vi "HAPS_main_Phase_Cali_Preamp.vi"() -> ()   [LabVIEW 2023, in "HAPS.lvlib"]
uses:
  HAPS.lvlib
  MCU_Function.ctl
  set_ele.ctl
  HAPS_SerialPort.ctl
  HAPS_MCU_ELE_Func.ctl
panel:
  in  "FileNote":string
  out "Array 2":dbl[](array[numeric])
  out "Array":i32[](array[numeric])
  out "ele_gain":i32
  out "comn_gain":i32
  out "Duration":dbl
  in  "Init?":bool
  out "In-Phase : Phase(degree)":dbl[](graph)
  out "In-Phase : Gain(dB)":dbl[](graph)
  out "channel":i32
  out "chain_id":i32
  out "group":i32
  out "array_id":i32
  in  "Phase diff. Criteria":dbl format="%#_13g"
  in  "Tx/Rx":enum16{"Rx", "Tx"}(ring)=enum."Tx"
  in  "array_id (MCU index)":i32
  in  "MCU_UART_addr":refnum<visa-resource-name>="COM1"
  in  "Max Steps":i32=10
  in  "Target(degree)":dbl format="%#_13g"
  in  "SweepPoints":i32=11
  in  "sParameter":i32=21
  in  "Stop_Freq(GHz)":dbl=39.5
  in  "Start_Freq(GHz)":dbl=38.5
  in  "VISA resource name":refnum<visa-resource-name>="TCPIP0::192.168.119.45::inst0::INSTR"
  in  "HAPS_Equipment":enum16{"Keysight", "R&S"}(ring)=enum."R&S"
  # "TCPIP0::169.254.52.242::hislip0::INSTR"
  # "TCPIP0::192.168.119.45::inst0::INSTR"
  # "HAPS_24x24_Phase_Calibration_Preamp"
  # "VNA"
  # "TCPIP0::192.168.1.31::hislip0::INSTR"
  # "Test Status"
  # "DUT"
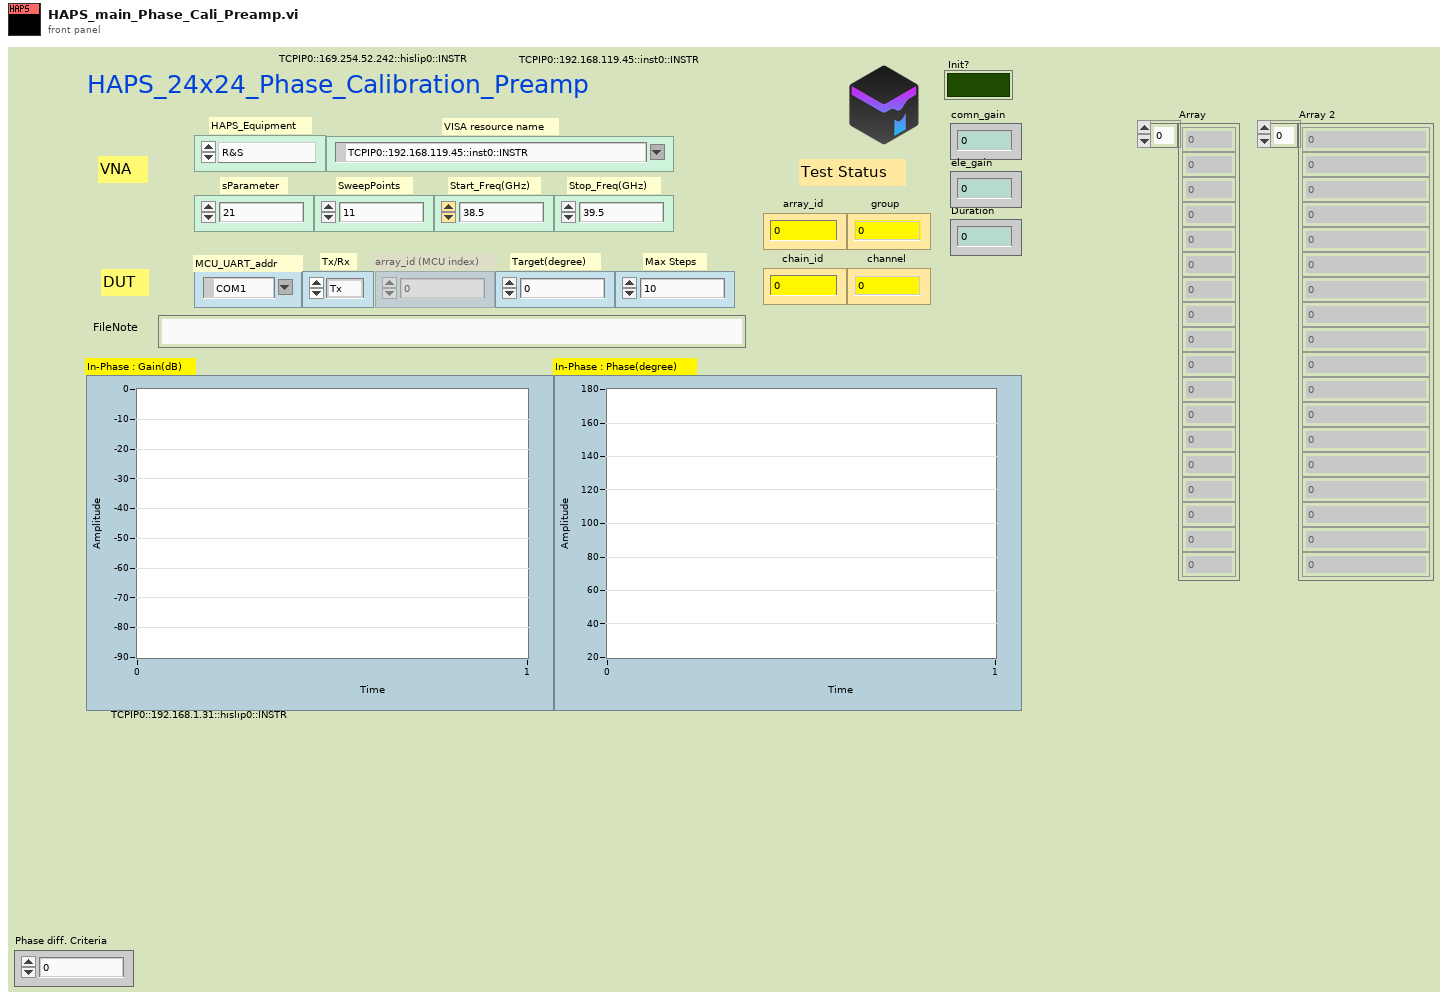
[diagram p1: front panel]
types:
  T1 = typedef "HAPS.lvlib/HAPS_SerialPort.ctl" = enum16{"Init", "Close", "CMD", "Flush"}
  T2 = typedef "HAPS.lvlib/HAPS_MCU_ELE_Func.ctl" = enum16{"array_init", "set_com_gain", "set_ch_gain_phase", "set_pd_range", "get_preamp_temp", "get_bfic_temp", "get_tx_pd", "ch_on", "ch_on_2", "ch_ctrl_all", "array_ctrl_src"}
  T3 = typedef "HAPS.lvlib/set_ele.ctl" = cluster{"ch":i32, "chain_id":i32, "group":i32, "array_id":i32, "ele_phase":i32, "ele_gain":i32, "com_gain":i32, "pd_range":i32}
  T4 = typedef "HAPS.lvlib/MCU_Function.ctl" = cluster{"Tx/Rx":enum16{"Rx", "Tx"}, "Enable?":enum16{"OFF", "On"}, "Source":enum16{"MCU", "ACU"}}
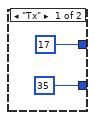
[diagram p2: hidden frame]
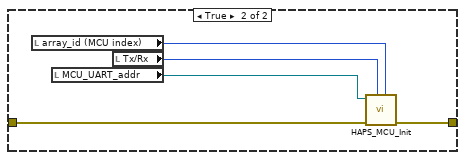
[diagram p3: hidden frame]
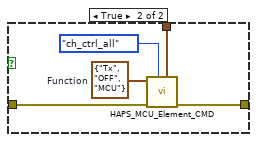
[diagram p6: hidden frame]
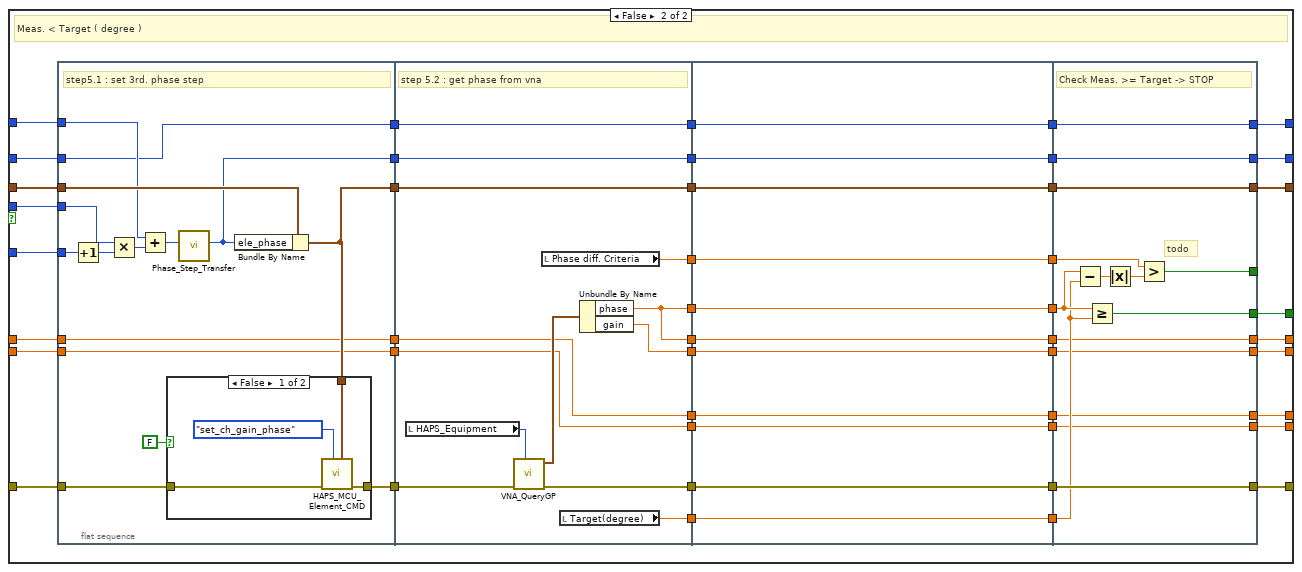
[diagram p11: hidden frame]
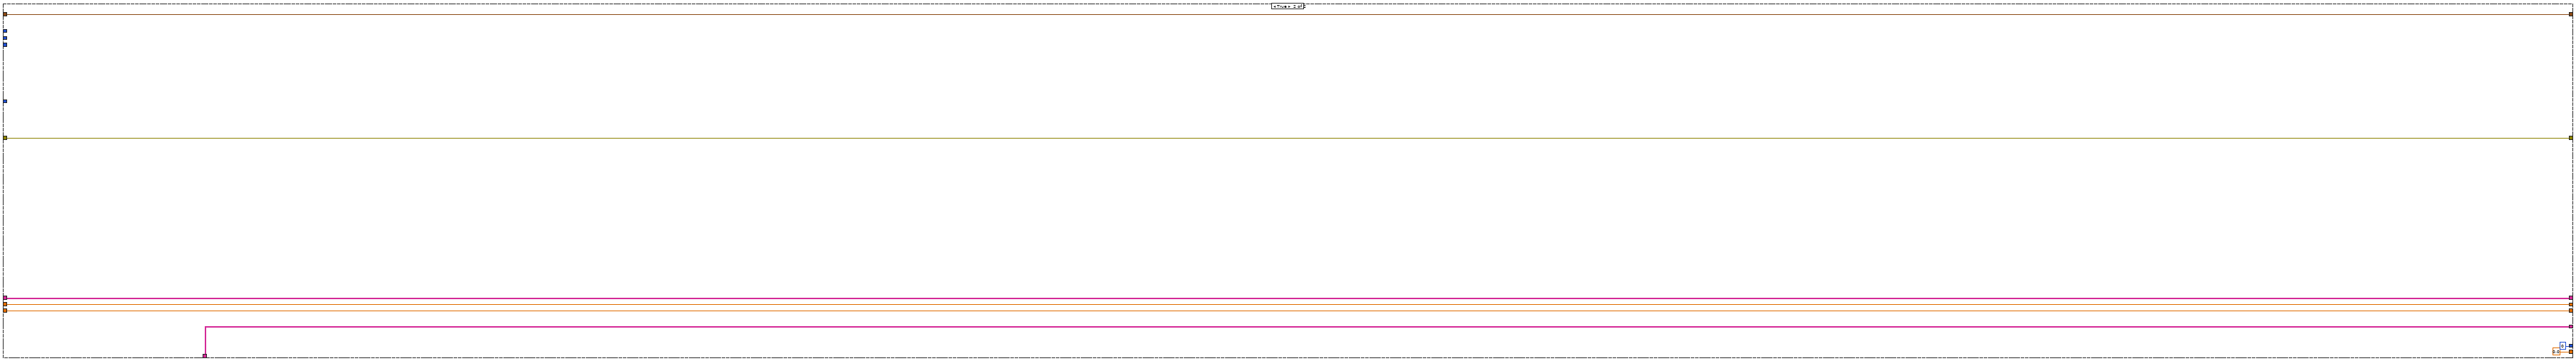
[diagram p13: hidden frame]
diagram:
  n1 = flat-sequence {
    tunnel: [w23] -> w16
    tunnel: [w30] -> w15
    tunnel: [errorcluster {"status"=FALSE, "code"=0, "source"=""} ("error in")] -> w13
    tunnel: ["sParameter"] -> w11
    tunnel: ["VISA resource name"] -> w10
    tunnel: ["Start_Freq(GHz)"] -> w9
    tunnel: ["Stop_Freq(GHz)"] -> w8
    tunnel: ["SweepPoints"] -> w7
    tunnel: ["HAPS_Equipment"] -> w6
    tunnel: [w20] -> w4
    tunnel: w16 -> [w47]
    tunnel: w15 -> [_]
    tunnel: [w47] -> w14
    tunnel: w13 -> [w46]
    tunnel: [w38] -> w12
    tunnel: w11 -> [w45]
    tunnel: w10 -> [w44]
    tunnel: w9 -> [w43]
    tunnel: w8 -> [w42]
    tunnel: w7 -> [w41]
    tunnel: w6 -> [w37]
    tunnel: [w35] -> w5
    tunnel: w4 -> [w35]
    tunnel: w14 -> [w67]
    tunnel: w12 -> [w68]
    tunnel: w5 -> [w64]
    tunnel: [w64] -> w3
    tunnel: [w63] -> w2
    tunnel: [w61] -> w1
    tunnel: [w631] -> _
    tunnel: w3 -> [w631]
    tunnel: w2 -> [w633]
    tunnel: w1 -> [w623]
    frame #0 {
      w21 = dbl[] []
      w23 = T3 {"ch"=0, "chain_id"=0, "group"=0, "array_id"=0, "ele_phase"=0, "ele_gain"=0, "com_gain"=0, "pd_range"=0}  # set_ele
      w30 = T4 {"Tx/Rx"=enum."Tx", "Enable?"=enum."OFF", "Source"=enum."MCU"}  # Function
      # "Init"
      n2 = case shown="\"Rx\"" "Tx/Rx" {
        tunnel: [17 ("comn_ele_gain") 17 ("comn_ele_gain")] -> w18
        tunnel: [35 ("comn_ele_gain") 22 ("comn_ele_gain")] -> w17
        frame "Tx" {
        }
        frame "Rx" {
        }
      }
      "comn_gain" <- w18
      "ele_gain" <- w17
      n3 = Get Date/Time In Seconds() -> (seconds since 1Jan1904=w20:timestamp)
      "In-Phase : Gain(dB)" <- w21
      "In-Phase : Phase(degree)" <- w21
    }
    frame #1 {
      # "settting before Calibration"
      n4 = call "VNA_init.vi"("Stop_Freq(GHz)"=w42, "HAPS_MCU_CMD"=w37, "Start_Freq(GHz)"=w43, "sParameter"=w45, "error in"=w46, "SweepPoints"=w41, "Mark no."=1, "VISA resource name"=w44) -> ("error out"=w39:errorcluster)  [unwired: 3 in]
      n5 = case shown="False" "Init?" {
        tunnel: w39 -> [w54 w59]
        tunnel: [w50 w58] -> w38
        frame False {
          n6 = local read "MCU_UART_addr"() -> (w52:refnum<visa-resource-name>)
          n7 = call "HAPS_MCU_SerialPort.vi"("HAPS_SerialPort_Func"=HAPS_SerialPort."Init", "error in"=w54, "VISA resource name"=w52) -> ("error out"=w51:errorcluster)  [unwired: 6 in, 2 out]
          n8 = call "HAPS_MCU_SerialPort.vi"("Command"="log_en 0", "HAPS_SerialPort_Func"=enum16{"Init", "Close", "CMD"}."CMD" ("HAPS_SerialPort"), "error in"=w51) -> ("error out"=w50:errorcluster)  [unwired: 6 in, 2 out]
        }
        frame True {
          n9 = local read "array_id (MCU index)"() -> (w56:i32)
          n10 = local read "MCU_UART_addr"() -> (w57:refnum<visa-resource-name>)
          n11 = local read "Tx/Rx"() -> (w55:enum16{"Rx", "Tx"})
          n12 = call "HAPS_MCU_Init.vi"("array_id"=w56, "Tx/Rx"=w55, "error in"=w59, "VISA resource name"=w57) -> ("error out"=w58:errorcluster)  [unwired: 7 in]
        }
      }
    }
    frame #2 {
      w60 = i32[][] [[2, 0, 0, 8, 8, 10, 11, 9, 9, 1, 1, 3], [3, 1, 1, 9, 9, 11, 13, 15, 15, 7, 7, 5], [5, 7, 7, 15, 15, 13, 14, 14, 6, 6, 4, 12]]  # Preamp_ch
      # "Calibration"
      n13 = for {
        N: 3 -> [_]
        shift-right: [w79] -> _
        shift-left: w67 -> [w75]
        shift-right: [w78] -> w63
        shift-left: string[][] [] -> [w73]
        shift-right: [w77] -> _
        shift-left: w68 -> [w76]
        shift-right: [w71] -> w61
        shift-left: string[][] [] -> [w72]
        tunnel: w60 -> [w70] mode=indexing
        i -> [w74]
        w69 = dbl[] []
        # "group ( 0~2 )"
        n14 = for {
          N: 12 -> [_]
          shift-right: [w95] -> w79
          shift-left: w75 -> [w91]
          shift-right: [w94] -> w78
          shift-left: w73 -> [w88]
          shift-right: [w93] -> w77
          shift-left: w76 -> [w92]
          tunnel: w74 -> [w90]
          shift-right: [w83] -> _
          shift-left: w69 -> [_]
          shift-right: [w83] -> _
          shift-left: w69 -> [_]
          shift-right: [w86] -> w71
          shift-left: w72 -> [w87]
          tunnel: w70 -> [w85] mode=indexing
          i -> [w89]
          w83 = dbl[] []
          w84 = dbl[] []
          # "Chain_id ( 0~11 )"
          n15 = for {
            N: 16 -> [_]
            shift-right: [w119] -> w95
            shift-left: w91 -> [w107]
            shift-right: [w117] -> w94
            shift-left: w88 -> [w118]
            shift-right: [w109] -> w93
            shift-left: w92 -> [w108]
            tunnel: w90 -> [w101]
            tunnel: w89 -> [w100]
            shift-right: [w114] -> _
            shift-left: w84 -> [w116]
            shift-right: [w113] -> _
            shift-left: w84 -> [w115]
            shift-right: [w111] -> w86
            shift-left: w87 -> [w112]
            tunnel: w85 -> [w106]
            tunnel: [w98] -> w82 mode=indexing
            tunnel: [w97] -> w81 mode=indexing
            i -> [w110]
            # "Channel ( 0~15 )"
            n16 = Equal?(x=2, y=w101) -> (x = y?=w105:bool)
            n17 = Equal?(x=11, y=w100) -> (x = y?=w104:bool)
            n18 = And(x=w105, y=w104) -> (x .and. y?=w99:bool)
            n19 = case shown="False" w99 {
              tunnel: [w120 w615] -> w119
              tunnel: w118 -> [w152 w617]
              tunnel: [w151 w617] -> w117
              tunnel: w116 -> [w150 w618]
              tunnel: w115 -> [w149 w619]
              tunnel: [w148 w618] -> w114
              tunnel: [w147 w619] -> w113
              tunnel: w112 -> [w146 w620]
              tunnel: [w145 w620] -> w111
              tunnel: w101 -> [w128 _]
              tunnel: w100 -> [w127 _]
              tunnel: w110 -> [w142 _]
              tunnel: [w140 w616] -> w109
              tunnel: w108 -> [w136 w616]
              tunnel: w107 -> [w134 w615]
              tunnel: w106 -> [w129 _]
              tunnel: [w122 0 ("Esitmation_Step")] -> w98
              tunnel: [w121 0.0 ("phase")] -> w97
              frame False {
                n20 = local read "array_id (MCU index)"() -> (w132:i32)
                n21 = Bundle By Name(cluster=w134, "array_id"=w132, "group"=3, "chain_id"=0, "ch"=w129) -> (w133:T3)
                n22 = call "HAPS_MCU_Element_CMD.vi"("set_ele"=w133, "HAPS_MCU_ELE_Func."=HAPS_MCU_ELE_Func."ch_on", "error in"=w136) -> ("error out"=w135:errorcluster)  [unwired: 7 in, 1 out]
                n23 = Bundle By Name(cluster=w134, "array_id"=w132, "group"=w128, "chain_id"=w127, "ch"=w142) -> (w141:T3)
                n24 = call "HAPS_MCU_Element_CMD.vi"("set_ele"=w141, "HAPS_MCU_ELE_Func."=HAPS_MCU_ELE_Func."ch_on", "error in"=w135) -> ("error out"=w143:errorcluster)  [unwired: 7 in, 1 out]
                n25 = flat-sequence {
                  tunnel: w141 -> [w229]
                  tunnel: w143 -> [w230]
                  tunnel: [w231] -> w207
                  tunnel: [w227] -> w206
                  tunnel: w142 -> [w226]
                  tunnel: [w225] -> w205
                  tunnel: w152 -> [w225]
                  tunnel: w128 -> [w223]
                  tunnel: w127 -> [w222]
                  tunnel: [w221] -> w204
                  tunnel: w150 -> [w221]
                  tunnel: [w220] -> w203
                  tunnel: w149 -> [w220]
                  tunnel: w146 -> [w219]
                  tunnel: [w219] -> w202
                  tunnel: w207 -> [w248]
                  tunnel: [w249] -> w201
                  tunnel: [w240] -> w200
                  tunnel: [w247] -> w199
                  tunnel: w206 -> [w247]
                  tunnel: [w244] -> w198
                  tunnel: w205 -> [w244]
                  tunnel: [w243] -> w197
                  tunnel: w204 -> [w243]
                  tunnel: [w242] -> w196
                  tunnel: w203 -> [w242]
                  tunnel: w202 -> [w241]
                  tunnel: [w241] -> w195
                  tunnel: [w240] -> w122
                  tunnel: [w239] -> w121
                  tunnel: w201 -> [w254]
                  tunnel: [w255] -> w194
                  tunnel: w200 -> [w260]
                  tunnel: [w260] -> w193
                  tunnel: w199 -> [w253]
                  tunnel: [w253] -> w192
                  tunnel: w198 -> [w259]
                  tunnel: [w259] -> w191
                  tunnel: w197 -> [w258]
                  tunnel: [w258] -> w190
                  tunnel: w196 -> [w257]
                  tunnel: [w257] -> w189
                  tunnel: w195 -> [w256]
                  tunnel: [w256] -> w188
                  tunnel: w194 -> [w275]
                  tunnel: w193 -> [w272]
                  tunnel: w192 -> [w274]
                  tunnel: [w276] -> w187
                  tunnel: [w273] -> w186
                  tunnel: [w272] -> w185
                  tunnel: [w271] -> w184
                  tunnel: w191 -> [w271]
                  tunnel: w190 -> [w270]
                  tunnel: w189 -> [w269]
                  tunnel: [w270] -> w183
                  tunnel: [w269] -> w182
                  tunnel: w188 -> [w268]
                  tunnel: [w268] -> w181
                  tunnel: w187 -> [w297]
                  tunnel: w186 -> [w290]
                  tunnel: [w298] -> w180
                  tunnel: [w292] -> w179
                  tunnel: [w291] -> w178
                  tunnel: [w290] -> w177
                  tunnel: [w289] -> w176
                  tunnel: w185 -> [w289]
                  tunnel: [w287] -> w175
                  tunnel: w184 -> [w287]
                  tunnel: [w286] -> w174
                  tunnel: w183 -> [w286]
                  tunnel: [w285] -> w173
                  tunnel: w182 -> [w285]
                  tunnel: w181 -> [w284]
                  tunnel: [w284] -> w172
                  tunnel: [w283] -> w126
                  tunnel: [w282] -> w124
                  tunnel: w180 -> [w302]
                  tunnel: [w303] -> w171
                  tunnel: w179 -> [w311]
                  tunnel: [w311] -> w170
                  tunnel: w178 -> [w310]
                  tunnel: [w310] -> w169
                  tunnel: w177 -> [w309]
                  tunnel: [w309] -> w168
                  tunnel: w176 -> [w308]
                  tunnel: [w308] -> w167
                  tunnel: w175 -> [w307]
                  tunnel: [w307] -> w166
                  tunnel: w174 -> [w306]
                  tunnel: [w306] -> w165
                  tunnel: w173 -> [w305]
                  tunnel: [w305] -> w164
                  tunnel: w172 -> [w304]
                  tunnel: [w304] -> w163
                  tunnel: w126 -> [w300]
                  tunnel: [w300] -> w125
                  tunnel: w124 -> [w299]
                  tunnel: [w299] -> w123
                  tunnel: w171 -> [w331]
                  tunnel: w170 -> [w332]
                  tunnel: w169 -> [w333]
                  tunnel: w168 -> [w334]
                  tunnel: w167 -> [w319]
                  tunnel: [w330] -> w162
                  tunnel: [w329] -> w161
                  tunnel: [w328] -> w160
                  tunnel: [w327] -> w159
                  tunnel: [w326] -> w158
                  tunnel: [w325] -> w157
                  tunnel: w166 -> [w325]
                  tunnel: [w324] -> w156
                  tunnel: w165 -> [w323]
                  tunnel: w164 -> [w322]
                  tunnel: [w323] -> w155
                  tunnel: [w322] -> w154
                  tunnel: w163 -> [w321]
                  tunnel: [w320] -> w153
                  tunnel: w125 -> [w318]
                  tunnel: w123 -> [w317]
                  tunnel: [w612] -> w120
                  tunnel: w162 -> [w612]
                  tunnel: w161 -> [w611]
                  tunnel: w160 -> [w583]
                  tunnel: w159 -> [w584]
                  tunnel: w158 -> [w606]
                  tunnel: w157 -> [w590]
                  tunnel: [w592] -> w151
                  tunnel: [w591] -> w139
                  tunnel: w156 -> [w591]
                  tunnel: w155 -> [w587]
                  tunnel: w154 -> [w586]
                  tunnel: [w589] -> w148
                  tunnel: [w588] -> w147
                  tunnel: w153 -> [w582]
                  tunnel: [w582] -> w145
                  frame #0 {
                    w232 = 0  # pd_range
                    w233 = 0  # Init_Phase_Step
                    # "step 1. : First get phase step \"0\" for element BFIC"
                    n26 = local read "array_id (MCU index)"() -> (w224:i32)
                    "array_id" <- w224
                    n27 = local read "ele_gain"() -> (w216:i32)
                    n28 = local read "comn_gain"() -> (w217:i32)
                    n29 = Bundle By Name(cluster=w229, "array_id"=w224, "group"=w223, "chain_id"=w222, "ch"=w226, "com_gain"=w217, "ele_gain"=w216, "ele_phase"=w233, "pd_range"=w232) -> (w227:T3)
                    n30 = case shown="False" FALSE {
                      tunnel: [w237 w238] -> w231
                      tunnel: w230 -> [w236 w238]
                      tunnel: HAPS_MCU_ELE_Func."set_ch_gain_phase" ("HAPS_MCU_ELE_Func.") -> [w235 _]
                      tunnel: w227 -> [w234 _]
                      frame False {
                        n31 = call "HAPS_MCU_Element_CMD.vi"("set_ele"=w234, "HAPS_MCU_ELE_Func."=w235, "error in"=w236) -> ("error out"=w237:errorcluster)  [unwired: 7 in, 1 out]
                      }
                      frame True {
                      }
                    }
                    "group" <- w223
                    "chain_id" <- w222
                    "channel" <- w226
                  }
                  frame #1 {
                    # "todo:gain"
                    # "step 2. : get first pahse data from vna"
                    n32 = local read "HAPS_Equipment"() -> (w245:enum16{"Keysight", "R&S"})
                    n33 = call "VNA_QueryGP.vi"("HAPS_Equipment"=w245, "error in"=w248) -> ("error out"=w249:errorcluster, "queryMarker"=w250:cluster{"gain":dbl, "phase":dbl})  [unwired: 8 in]
                    n34 = Unbundle By Name(w247) -> ("ele_phase"=w246:i32)
                    n35 = local read "Target(degree)"() -> (w251:dbl)
                    n36 = Unbundle By Name(w250) -> ("phase"=w239:dbl)  [unwired: 1 out]
                    n37 = call "Estimation_Steps.vi"("Target(degree)"=w251, "Source_Phase_Step"=w246, "Input_Phase(degree)"=w239) -> ("Esitmation_Step"=w240:i32)  [unwired: 7 in, 1 out]
                  }
                  frame #2 {
                    n38 = case shown="False" FALSE {
                      tunnel: [w261 w266] -> w255
                      tunnel: w254 -> [w261 w265]
                      tunnel: w253 -> [_ w263]
                      frame False {
                      }
                      frame True {
                        w262 = T4 {"Tx/Rx"=enum."Tx", "Enable?"=enum."OFF", "Source"=enum."MCU"}  # Function
                        n39 = call "HAPS_MCU_Element_CMD.vi"("set_ele"=w263, "HAPS_MCU_ELE_Func."=HAPS_MCU_ELE_Func."ch_ctrl_all", "error in"=w265, "Function"=w262) -> ("error out"=w266:errorcluster)  [unwired: 6 in, 1 out]
                      }
                    }
                  }
                  frame #3 {
                    # "source.\nphase step"
                    # "step 3.  set estimation phase step in second time"
                    n40 = Bundle By Name(cluster=w274, "ele_phase"=w272) -> (w273:T3)
                    n41 = case shown="False" FALSE {
                      tunnel: [w280 w281] -> w276
                      tunnel: w275 -> [w279 w281]
                      tunnel: w273 -> [w278 _]
                      frame False {
                        n42 = call "HAPS_MCU_Element_CMD.vi"("set_ele"=w278, "HAPS_MCU_ELE_Func."=HAPS_MCU_ELE_Func."set_ch_gain_phase", "error in"=w279) -> ("error out"=w280:errorcluster)  [unwired: 7 in, 1 out]
                      }
                      frame True {
                      }
                    }
                  }
                  frame #4 {
                    # "todo:gain"
                    # "step 4. : get second time pahse from vna"
                    n43 = local read "HAPS_Equipment"() -> (w288:enum16{"Keysight", "R&S"})
                    n44 = call "VNA_QueryGP.vi"("HAPS_Equipment"=w288, "error in"=w297) -> ("error out"=w298:errorcluster, "queryMarker"=w293:cluster{"gain":dbl, "phase":dbl})  [unwired: 8 in]
                    n45 = Unbundle By Name(w293) -> ("phase"=w283:dbl, "gain"=w282:dbl)
                    n46 = local read "Target(degree)"() -> (w294:dbl)
                    n47 = Greater Or Equal?(x=w283, y=w294) -> (x >= y?=w292:bool)
                    n48 = Select(t=1, s=w292, f=-1) -> (s? t:f=w291:i32)
                  }
                  frame #5 {
                    n49 = case shown="True" FALSE {
                      tunnel: [w312 w314] -> w303
                      tunnel: w302 -> [w312 w313]
                      frame False {
                      }
                      frame True {
                        w316 = T4 {"Tx/Rx"=enum."Tx", "Enable?"=enum."OFF", "Source"=enum."MCU"}  # Function
                        n50 = call "HAPS_MCU_Element_CMD.vi"("HAPS_MCU_ELE_Func."=HAPS_MCU_ELE_Func."ch_ctrl_all", "error in"=w313, "Function"=w316) -> ("error out"=w314:errorcluster)  [unwired: 7 in, 1 out]
                      }
                    }
                  }
                  frame #6 {
                    # "source.\nphase step"
                    # "Mea. >= Target"
                    # "source.\ndegree"
                    # "step 5. : find in-phase step"
                    n51 = for {
                      N: "Max Steps" -> [_]
                      shift-right: [w368] -> w330
                      shift-left: w334 -> [w371]
                      shift-right: [w369] -> w324
                      shift-left: w331 -> [w374]
                      shift-right: [w336] -> w326
                      shift-left: w319 -> [w370]
                      tunnel: w332 -> [w375]
                      tunnel: w333 -> [w372]
                      shift-right: [w343] -> w329
                      shift-left: _ -> [_]
                      shift-right: [w340] -> w327
                      shift-left: w318 -> [w348]
                      shift-right: [w339] -> w328
                      shift-left: w317 -> [w347]
                      shift-right: [w350] -> w320
                      shift-left: w321 -> [w352]
                      tunnel: w319 -> [w349]
                      i -> [w373]
                      stop <- w343 stop-if-true
                      n52 = case shown="True" w375 {
                        tunnel: w374 -> [w429 w522]
                        tunnel: w373 -> [w428 w521]
                        tunnel: w372 -> [w427 w520]
                        tunnel: w371 -> [w426 w519]
                        tunnel: w370 -> [w425 w518]
                        tunnel: [w424 w517] -> w369
                        tunnel: [w423 w516] -> w368
                        tunnel: [w422 w515] -> w338
                        tunnel: [w414 w511] -> w346
                        tunnel: [w411 w510] -> w345
                        tunnel: [w410 w509] -> w342
                        tunnel: [w407 w508] -> w344
                        tunnel: [w406 w507] -> w341
                        tunnel: w349 -> [w405 w506]
                        tunnel: w348 -> [w402 w484]
                        tunnel: w347 -> [w400 w482]
                        tunnel: [w398 w489] -> w337
                        frame True {
                          # "New"
                          # "Last"
                          # "Meas. >= Target ( degree )"
                          n53 = flat-sequence {
                            tunnel: w429 -> [w441]
                            tunnel: w428 -> [w444]
                            tunnel: w427 -> [w443]
                            tunnel: w426 -> [w438]
                            tunnel: w425 -> [w430]
                            tunnel: [w442] -> w421
                            tunnel: [w439] -> w420
                            tunnel: [w435] -> w419
                            tunnel: w405 -> [w431]
                            tunnel: [w433] -> w403
                            tunnel: w402 -> [w433]
                            tunnel: [w432] -> w401
                            tunnel: w400 -> [w432]
                            tunnel: [w430] -> w396
                            tunnel: w421 -> [w459]
                            tunnel: w420 -> [w462]
                            tunnel: w419 -> [w461]
                            tunnel: [w460] -> w418
                            tunnel: [w462] -> w417
                            tunnel: [w461] -> w416
                            tunnel: [w456] -> w415
                            tunnel: [w457] -> w413
                            tunnel: [w453] -> w412
                            tunnel: [w455] -> w409
                            tunnel: [w456] -> w408
                            tunnel: [w452] -> w404
                            tunnel: w403 -> [w452]
                            tunnel: w401 -> [w451]
                            tunnel: [w451] -> w399
                            tunnel: [w450] -> w397
                            tunnel: w396 -> [w450]
                            tunnel: [w475] -> w414
                            tunnel: [w474] -> w422
                            tunnel: [w476] -> w423
                            tunnel: [w477] -> w424
                            tunnel: w418 -> [w477]
                            tunnel: w417 -> [w476]
                            tunnel: w416 -> [w474]
                            tunnel: w415 -> [w473]
                            tunnel: w413 -> [w471]
                            tunnel: w412 -> [w469]
                            tunnel: [w468] -> _
                            tunnel: [w467] -> w411
                            tunnel: [w465] -> w410
                            tunnel: w409 -> [w465]
                            tunnel: w408 -> [w467]
                            tunnel: [w466] -> w407
                            tunnel: [w464] -> w406
                            tunnel: w404 -> [w466]
                            tunnel: w399 -> [w464]
                            tunnel: [w463] -> w398
                            tunnel: w397 -> [w463]
                            frame #0 {
                              # "step5.1 : set 3rd. phase step"
                              n54 = Increment(x=w444) -> (x+1=w440:i32)
                              n55 = Multiply(x=w443, y=w440) -> (x*y=w437:i32)
                              n56 = Add(x=w431, y=w437) -> (x+y=w436:i32)
                              n57 = call "Phase_Step_Transfer.vi"("Input_Phase_Step"=w436) -> ("Output_Phase_Step"=w435:i32)  [unwired: 10 in]
                              n58 = Bundle By Name(cluster=w438, "ele_phase"=w435) -> (w439:T3)
                              n59 = case shown="False" FALSE {
                                tunnel: [w448 w449] -> w442
                                tunnel: w441 -> [w447 w449]
                                tunnel: w439 -> [w446 _]
                                frame False {
                                n60 = call "HAPS_MCU_Element_CMD.vi"("set_ele"=w446, "HAPS_MCU_ELE_Func."=HAPS_MCU_ELE_Func."set_ch_gain_phase", "error in"=w447) -> ("error out"=w448:errorcluster)  [unwired: 7 in, 1 out]
                                }
                                frame True {
                                }
                              }
                            }
                            frame #1 {
                              # "step 5.2 : get phase from vna"
                              n61 = local read "HAPS_Equipment"() -> (w454:enum16{"Keysight", "R&S"})
                              n62 = call "VNA_QueryGP.vi"("HAPS_Equipment"=w454, "error in"=w459) -> ("error out"=w460:errorcluster, "queryMarker"=w458:cluster{"gain":dbl, "phase":dbl})  [unwired: 8 in]
                              n63 = local read "Phase diff. Criteria"() -> (w453:dbl)
                              n64 = local read "Target(degree)"() -> (w457:dbl)
                              n65 = Unbundle By Name(w458) -> ("phase"=w456:dbl, "gain"=w455:dbl)
                            }
                            frame #2 {
                              # "todo"
                              # "Check Meas. <= Target => STOP"
                              n66 = Subtract(x=w473, y=w471) -> (x-y=w472:dbl)
                              n67 = Less Or Equal?(x=w473, y=w471) -> (x <= y?=w475:bool)
                              n68 = Absolute Value(x=w472) -> (abs(x)=w470:dbl)
                              n69 = Greater?(x=w469, y=w470) -> (0:w468:bool)
                            }
                          }
                        }
                        frame False {
                          # "Meas. < Target ( degree )"
                          n70 = flat-sequence {
                            tunnel: w522 -> [w534]
                            tunnel: w521 -> [w537]
                            tunnel: w520 -> [w536]
                            tunnel: w519 -> [w531]
                            tunnel: w518 -> [w523]
                            tunnel: [w535] -> w514
                            tunnel: [w532] -> w513
                            tunnel: [w528] -> w512
                            tunnel: w506 -> [w526]
                            tunnel: [w523] -> w486
                            tunnel: [w525] -> w485
                            tunnel: w484 -> [w525]
                            tunnel: [w524] -> w483
                            tunnel: w482 -> [w524]
                            tunnel: w514 -> [w552]
                            tunnel: w513 -> [w555]
                            tunnel: w512 -> [w554]
                            tunnel: [w553] -> w505
                            tunnel: [w555] -> w503
                            tunnel: [w554] -> w501
                            tunnel: [w549] -> w499
                            tunnel: [w550] -> w497
                            tunnel: [w546] -> w495
                            tunnel: [w548] -> w493
                            tunnel: [w549] -> w491
                            tunnel: [w545] -> w487
                            tunnel: w486 -> [w545]
                            tunnel: w485 -> [w544]
                            tunnel: w483 -> [w543]
                            tunnel: [w544] -> w480
                            tunnel: [w543] -> w478
                            tunnel: w505 -> [w559]
                            tunnel: [w559] -> w504
                            tunnel: w503 -> [w566]
                            tunnel: [w566] -> w502
                            tunnel: w501 -> [w565]
                            tunnel: [w565] -> w500
                            tunnel: w499 -> [w564]
                            tunnel: [w564] -> w498
                            tunnel: w497 -> [w563]
                            tunnel: [w563] -> w496
                            tunnel: w495 -> [w562]
                            tunnel: [w562] -> w494
                            tunnel: w493 -> [w561]
                            tunnel: [w561] -> w492
                            tunnel: w491 -> [w560]
                            tunnel: [w560] -> w490
                            tunnel: [w558] -> w488
                            tunnel: w487 -> [w558]
                            tunnel: [w557] -> w481
                            tunnel: w480 -> [w557]
                            tunnel: [w556] -> w479
                            tunnel: w478 -> [w556]
                            tunnel: [w579] -> w511
                            tunnel: [w578] -> w515
                            tunnel: [w580] -> w516
                            tunnel: [w581] -> w517
                            tunnel: w504 -> [w581]
                            tunnel: w502 -> [w580]
                            tunnel: w500 -> [w578]
                            tunnel: w498 -> [w577]
                            tunnel: w496 -> [w575]
                            tunnel: w494 -> [w573]
                            tunnel: [w572] -> _
                            tunnel: [w570] -> w510
                            tunnel: [w568] -> w509
                            tunnel: w492 -> [w568]
                            tunnel: w490 -> [w570]
                            tunnel: [w569] -> w508
                            tunnel: [w567] -> w507
                            tunnel: [w571] -> w489
                            tunnel: w488 -> [w571]
                            tunnel: w481 -> [w569]
                            tunnel: w479 -> [w567]
                            frame #0 {
                              # "step5.1 : set 3rd. phase step"
                              n71 = Increment(x=w537) -> (x+1=w533:i32)
                              n72 = Multiply(x=w536, y=w533) -> (x*y=w530:i32)
                              n73 = Add(x=w526, y=w530) -> (x+y=w529:i32)
                              n74 = call "Phase_Step_Transfer.vi"("Input_Phase_Step"=w529) -> ("Output_Phase_Step"=w528:i32)  [unwired: 10 in]
                              n75 = Bundle By Name(cluster=w531, "ele_phase"=w528) -> (w532:T3)
                              n76 = case shown="False" FALSE {
                                tunnel: [w541 w542] -> w535
                                tunnel: w534 -> [w540 w542]
                                tunnel: w532 -> [w539 _]
                                frame False {
                                n77 = call "HAPS_MCU_Element_CMD.vi"("set_ele"=w539, "HAPS_MCU_ELE_Func."=HAPS_MCU_ELE_Func."set_ch_gain_phase", "error in"=w540) -> ("error out"=w541:errorcluster)  [unwired: 7 in, 1 out]
                                }
                                frame True {
                                }
                              }
                            }
                            frame #1 {
                              # "step 5.2 : get phase from vna"
                              n78 = local read "HAPS_Equipment"() -> (w547:enum16{"Keysight", "R&S"})
                              n79 = call "VNA_QueryGP.vi"("HAPS_Equipment"=w547, "error in"=w552) -> ("error out"=w553:errorcluster, "queryMarker"=w551:cluster{"gain":dbl, "phase":dbl})  [unwired: 8 in]
                              n80 = local read "Phase diff. Criteria"() -> (w546:dbl)
                              n81 = local read "Target(degree)"() -> (w550:dbl)
                              n82 = Unbundle By Name(w551) -> ("phase"=w549:dbl, "gain"=w548:dbl)
                            }
                            frame #2 {
                            }
                            frame #3 {
                              # "todo"
                              # "Check Meas. >= Target -> STOP"
                              n83 = Subtract(x=w577, y=w575) -> (x-y=w576:dbl)
                              n84 = Greater Or Equal?(x=w577, y=w575) -> (x >= y?=w579:bool)
                              n85 = Absolute Value(x=w576) -> (abs(x)=w574:dbl)
                              n86 = Greater?(x=w573, y=w574) -> (0:w572:bool)
                            }
                          }
                        }
                      }
                      n87 = property on="Tx/Rx" class="Enum (strict)"() -> ("RingText.Text"=w363:string)  [unwired: 2 in, 2 out]
                      n88 = local read "chain_id"() -> (w366:i32)
                      n89 = local read "array_id"() -> (w364:i32)
                      n90 = local read "channel"() -> (w367:i32)
                      n91 = local read "group"() -> (w365:i32)
                      n92 = case shown="True" w346 {
                        selector: w346 -> [w379 w395]
                        tunnel: w345 -> [w378 w389]
                        tunnel: w344 -> [_ w388]
                        tunnel: [w379 w395] -> w343
                        tunnel: w342 -> [w377 w387]
                        tunnel: w341 -> [_ w386]
                        tunnel: [w378 w385] -> w340
                        tunnel: [w377 w384] -> w339
                        tunnel: w338 -> [w376 w381]
                        tunnel: w337 -> [_ w382]
                        tunnel: [w376 w380] -> w336
                        frame False {
                        }
                        frame True {
                          n93 = local read "Target(degree)"() -> (w394:dbl)
                          n94 = Subtract(x=w389, y=w394) -> (x-y=w393:dbl)
                          n95 = Subtract(x=w388, y=w394) -> (x-y=w392:dbl)
                          n96 = Absolute Value(x=w393) -> (abs(x)=w391:dbl)
                          n97 = Absolute Value(x=w392) -> (abs(x)=w390:dbl)
                          n98 = Greater?(x=w391, y=w390) -> (0:w383:bool)
                          n99 = Select(t=w388, s=w383, f=w389) -> (s? t:f=w385:dbl)
                          n100 = Select(t=w382, s=w383, f=w381) -> (s? t:f=w380:i32)
                          n101 = Select(t=w386, s=w383, f=w387) -> (s? t:f=w384:dbl)
                        }
                      }
                      n102 = Number To Decimal String(number=w364) -> (decimal integer string=w362:string)  [unwired: 1 in]
                      n103 = Number To Decimal String(number=w365) -> (decimal integer string=w361:string)  [unwired: 1 in]
                      n104 = Number To Decimal String(number=w366) -> (decimal integer string=w360:string)  [unwired: 1 in]
                      n105 = Number To Decimal String(number=w367) -> (decimal integer string=w359:string)  [unwired: 1 in]
                      n106 = Number To Decimal String(number=w338) -> (decimal integer string=w358:string)  [unwired: 1 in]
                      n107 = Number To Fractional String(number=w345, precision (6)=i16 3) -> (F-format string=w355:string)  [unwired: 2 in]
                      n108 = Number To Fractional String(number=w342, precision (6)=i16 3) -> (F-format string=w354:string)  [unwired: 2 in]
                      n109 = Build Array(w363, w362, w361, w360, w359, w358, w355, w354, "log") -> (w351:string[])
                      n110 = Build Array (concatenate)(w352, w351) -> (w350:string[][])
                    }
                  }
                  frame #7 {
                    # "Result Update"
                    n111 = property on="Tx/Rx" class="Enum (strict)"() -> ("RingText.Text"=w599:string)  [unwired: 2 in, 2 out]
                    n112 = local read "chain_id"() -> (w608:i32)
                    n113 = local read "array_id"() -> (w610:i32)
                    n114 = local read "channel"() -> (w607:i32)
                    n115 = local read "group"() -> (w609:i32)
                    n116 = Build Array (concatenate)(w587, w583) -> (w589:dbl[])
                    n117 = Build Array (concatenate)(w586, w584) -> (w588:dbl[])
                    n118 = Select(t="Pass", s=w611, f="Failure") -> (s? t:f=w593:string)
                    n119 = local write "In-Phase : Phase(degree)"(w588) -> ()
                    n120 = local write "In-Phase : Gain(dB)"(w589) -> ()
                    n121 = Number To Fractional String(number=w584, precision (6)=i16 3) -> (F-format string=w595:string)  [unwired: 2 in]
                    n122 = Number To Decimal String(number=w610) -> (decimal integer string=w601:string)  [unwired: 1 in]
                    n123 = Number To Decimal String(number=w609) -> (decimal integer string=w600:string)  [unwired: 1 in]
                    n124 = Number To Decimal String(number=w608) -> (decimal integer string=w598:string)  [unwired: 1 in]
                    n125 = Number To Decimal String(number=w607) -> (decimal integer string=w597:string)  [unwired: 1 in]
                    n126 = Number To Decimal String(number=w606) -> (decimal integer string=w596:string)  [unwired: 1 in]
                    n127 = Number To Fractional String(number=w583, precision (6)=i16 3) -> (F-format string=w594:string)  [unwired: 2 in]
                    n128 = Build Array(w599, w601, w600, w598, w597, w596, w595, w594, w593) -> (w585:string[])
                    n129 = Build Array (concatenate)(w590, w585) -> (w592:string[][])
                  }
                }
                n130 = case shown="True" TRUE {
                  tunnel: [w208 w215] -> w140
                  tunnel: w139 -> [w208 w214]
                  tunnel: w120 -> [_ w212]
                  frame False {
                  }
                  frame True {
                    w213 = T4 {"Tx/Rx"=enum."Tx", "Enable?"=enum."OFF", "Source"=enum."MCU"}  # Function
                    n131 = Bundle By Name(cluster=w213, "Enable?"=enum16{"OFF", "On"}."OFF") -> (w210:T4)
                    n132 = call "HAPS_MCU_Element_CMD.vi"("set_ele"=w212, "HAPS_MCU_ELE_Func."=HAPS_MCU_ELE_Func."ch_ctrl_all", "error in"=w214, "Function"=w210) -> ("error out"=w215:errorcluster)  [unwired: 6 in, 1 out]
                  }
                }
              }
              frame True {
              }
            }
          }
          "Array" <- w82
          "Array 2" <- w81
        }
      }
    }
    frame #3 {
      n133 = Get Date/Time In Seconds() -> (seconds since 1Jan1904=w632:timestamp)
      n134 = Subtract(x=w632, y=w631) -> (x-y=→"Duration":dbl)
      n135 = local read "array_id"() -> (w627:i32)
      n136 = local read "array_id"() -> (w636:i32)
      n137 = property on="Tx/Rx" class="Enum (strict)"() -> ("RingText.Text"=w628:string)  [unwired: 2 in, 2 out]
      n138 = local read "FileNote"() -> (w621:string)
      n139 = property on="Tx/Rx" class="Enum (strict)"() -> ("RingText.Text"=w635:string)  [unwired: 2 in, 2 out]
      n140 = property on="MCU_UART_addr" class="VISAName"() -> ("Text.Text"=w625:string)  [unwired: 2 in, 2 out]
      n141 = local read "FileNote"() -> (w622:string)
      n142 = property on="MCU_UART_addr" class="VISAName"() -> ("Text.Text"=w639:string)  [unwired: 2 in, 2 out]
      n143 = Number To Decimal String(number=w627) -> (decimal integer string=w626:string)  [unwired: 1 in]
      n144 = Number To Decimal String(number=w636) -> (decimal integer string=w637:string)  [unwired: 1 in]
      n145 = Format Into String(format string="HAPS_Phase_Cali_%s_MCU%s_%s_%s_DetailALL", w628, w626, w625, w621) -> (resulting string=w624:string)  [unwired: 2 in, 1 out]
      n146 = Format Into String(format string="HAPS_Phase_Cali_%s_MCU%s_%s_%s", w635, w637, w639, w622) -> (resulting string=w638:string)  [unwired: 2 in, 1 out]
      n147 = call "_save_csv_HAPS_MCU_PhaseCali.vi"("NoteName"=w624, "array in"=w623) -> ()  [unwired: 9 in, 1 out]
      n148 = call "_save_csv_HAPS_MCU_PhaseCali.vi"("NoteName"=w638, "array in"=w633) -> ()  [unwired: 9 in, 1 out]
    }
  }
